vi "Update Table.vi"(7 "Limit (10k)":i32=10000 format="%.0p", 8 "error in":errorcluster, 9 "Status Message Ref":refnum<vi>, 10 "Table Ref":refnum<vi>, 11 "New Data in":string[][](array[string])) -> (0 "error out":errorcluster, 3 "Table Data out":string[][](array[string]))   [LabVIEW 2025, in "Automotive Ethernet Bus Monitor UI.lvlib"]
doc: "Update the table data with new packages. Returns the whole updated data what can be set later."
uses:
  Automotive Ethernet Bus Monitor UI.lvlib
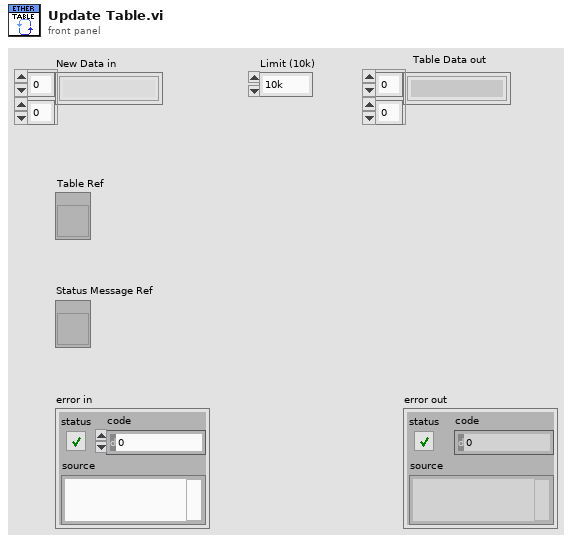
[diagram p1: front panel]
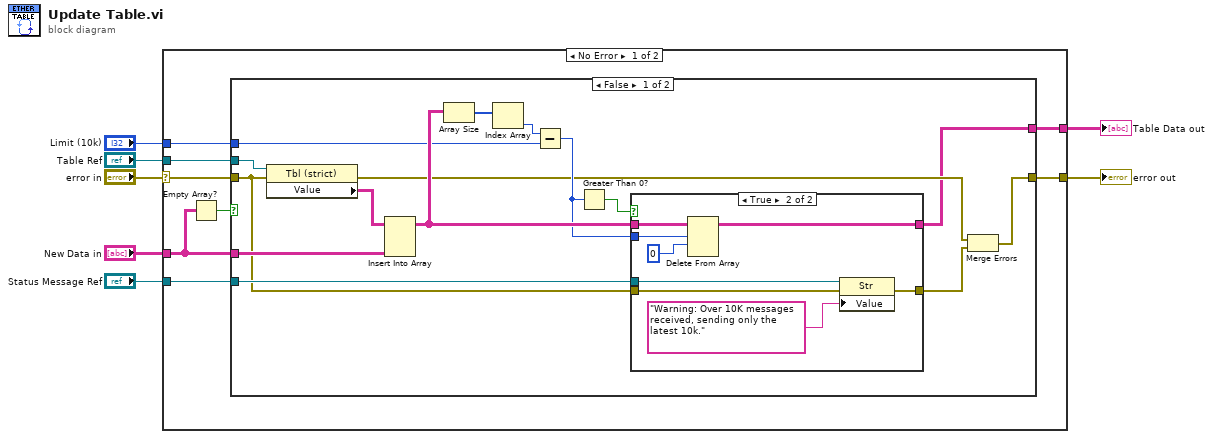
[diagram p0: block diagram]
diagram:
  n1 = case shown="No Error" "error in" {
    selector: "error in" -> [w14 w44]
    tunnel: "Table Ref" -> [w15 _]
    tunnel: "New Data in" -> [w11 w43]
    tunnel: [w13 w44] -> w4
    tunnel: "Limit (10k)" -> [w10 _]
    tunnel: "Status Message Ref" -> [w9 _]
    tunnel: [w8 w43] -> w1
    frame No Error {
      n2 = Empty Array?(array=w11) -> (empty?=w12:bool)
      n3 = case shown="False" w12 {
        tunnel: w11 -> [w28 w41]
        tunnel: w15 -> [w30 _]
        tunnel: w14 -> [w19 w42]
        tunnel: [w18 w42] -> w13
        tunnel: w10 -> [w25 _]
        tunnel: w9 -> [w21 _]
        tunnel: [w16 w41] -> w8
        frame False {
          n4 = property on="Property Node" class="Tbl (strict)"(reference=w30, error in=w19) -> (error out=w17:errorcluster, "Value"=w29:string[][])  [unwired: 1 out]
          n5 = Insert Into Array(array=w29, new element=w28) -> (w27:string[][])  [unwired: 2 in]
          n6 = Array Size(array=w27) -> (size(s)=w26:i32[])
          n7 = Index Array(array=w26) -> (element=w22:i32)  [unwired: 1 in]
          n8 = Subtract(x=w22, y=w25) -> (x-y=w23:i32)
          n9 = Greater Than 0?(x=w23) -> (x > 0?=w24:bool)
          n10 = case shown="True" w24 {
            tunnel: w27 -> [w32 w40]
            tunnel: [w32 w39] -> w16
            tunnel: w23 -> [_ w38]
            tunnel: w21 -> [_ w36]
            tunnel: [w31 w34] -> w20
            tunnel: w19 -> [w31 w33]
            frame False {
            }
            frame True {
              n11 = Delete From Array(array=w40, length=w38, index (row)=0) -> (array with subset deleted=w39:string[][])  [unwired: 1 in, 1 out]
              n12 = property on="Property Node" class="Str"(reference=w36, error in=w33, "Value"="Warning: Over 10K messages received, sending only the latest 10k.") -> (error out=w34:errorcluster)  [unwired: 1 out]
            }
          }
          n13 = Merge Errors(w17, w20) -> (w18:errorcluster)
        }
        frame True {
        }
      }
    }
    frame Error {
    }
  }
  "error out" <- w4
  "Table Data out" <- w1
